vi "Close UDP AND TCP connections.vi"(4 "error in":errorcluster, 6 "appended array 2":refnum<vi>[](array[refnum]), 7 "appended array":variant[](array[variant])) -> ()   [LabVIEW 2013]
panel:
  out "Array":refnum<k5>[](array[refnum])
  out "error out":errorcluster
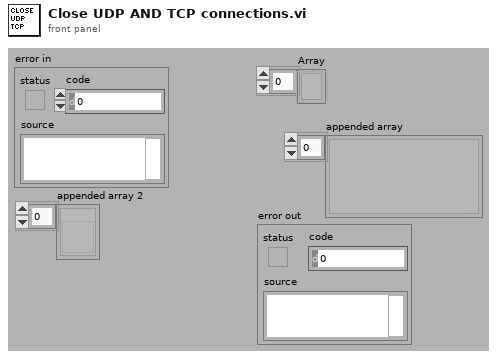
[diagram p1: front panel]
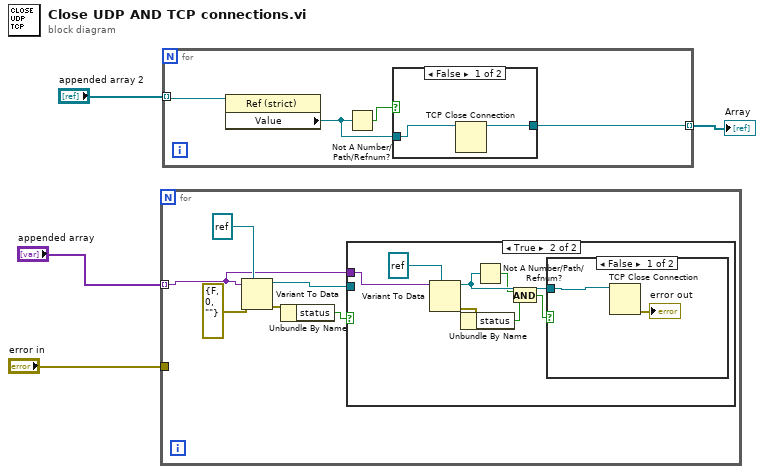
[diagram p0: block diagram]
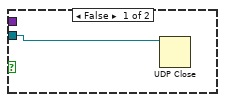
[diagram p3: hidden frame]
diagram:
  n1 = for {
    tunnel: "appended array" -> [w5] mode=indexing
    tunnel: "error in" -> [_]
    n2 = Variant To Data(error in=errorcluster {"status"=FALSE, "code"=0, "source"=""}, type=refnum<k16> refnum ("connection ID"), Variant=w5) -> (data=w6:refnum<k16>, error out=w8:errorcluster)
    n3 = Unbundle By Name(w8) -> ("status"=w7:bool)
    n4 = case shown="True" w7 {
      tunnel: w6 -> [w11 _]
      tunnel: w5 -> [_ w18]
      frame False {
        n5 = UDP Close(connection ID=w11) -> ()  [unwired: 1 in, 2 out]
      }
      frame True {
        n6 = Variant To Data(type=refnum<k5> refnum ("connection ID"), Variant=w18) -> (data=w15:refnum<k5>, error out=w16:errorcluster)  [unwired: 1 in]
        n7 = Unbundle By Name(w16) -> ("status"=w14:bool)
        n8 = Not A Number/Path/Refnum?(number/path/refnum=w15) -> (NaN/Path/Refnum?=w13:bool)
        n9 = And(x=w13, y=w14) -> (x .and. y?=w12:bool)
        n10 = case shown="False" w12 {
          tunnel: w15 -> [w20 _]
          frame False {
            n11 = TCP Close Connection(connection ID=w20) -> (error out=→"error out":errorcluster)  [unwired: 2 in, 1 out]
          }
          frame True {
          }
        }
      }
    }
  }
  n12 = for {
    tunnel: "appended array 2" -> [w24] mode=indexing
    tunnel: [w21] -> w1 mode=indexing
    n13 = property class="Ref (strict)"(reference=w24) -> ("Value"=w22:refnum<k5>)  [unwired: 1 in, 2 out]
    n14 = Not A Number/Path/Refnum?(number/path/refnum=w22) -> (NaN/Path/Refnum?=w23:bool)
    n15 = case shown="False" w23 {
      tunnel: w22 -> [w26 w27]
      tunnel: [w25 w27] -> w21
      frame False {
        n16 = TCP Close Connection(connection ID=w26) -> (connection ID out=w25:refnum<k5>)  [unwired: 2 in, 1 out]
      }
      frame True {
      }
    }
  }
  "Array" <- w1
